vi "SplitString.vi"(8 "error in (no error)":errorcluster, 11 "String in":string) -> (0 "error out":errorcluster, 2 "Array":string[](array[string]), 3 "String out":string)   [LabVIEW 2012]
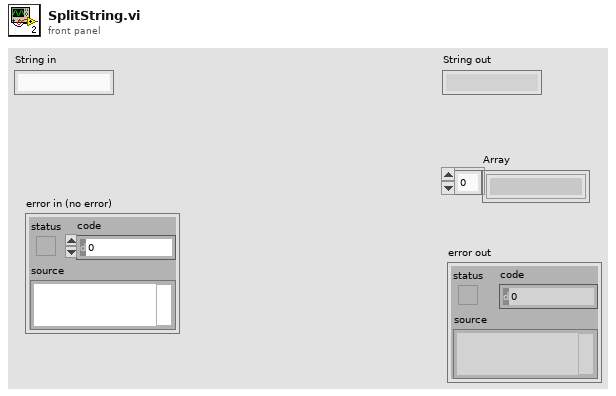
[diagram p1: front panel]
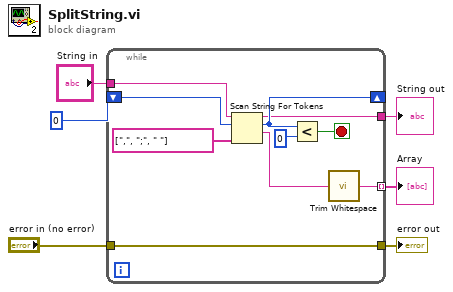
[diagram p0: block diagram]
diagram:
  n1 = while {
    shift-right: [w14] -> _
    shift-left: 0 -> [w16]
    tunnel: "String in" -> [w12]
    tunnel: [w9] -> w3 mode=indexing
    tunnel: "error in (no error)" -> [w8]
    tunnel: [w8] -> w4
    tunnel: [w7] -> w2
    stop <- w13 stop-if-true
    n2 = Scan String For Tokens(6:string[] [",", ";", " "], 8:w16, 9:w12) -> (1:w10:string, 2:w14:i32, 3:w7:string)  [unwired: 3 in, 1 out]
    n3 = Less?(x=w14, y=0) -> (x < y?=w13:bool)
    n4 = call <vilib>:"Trim Whitespace.vi"("string"=w10) -> ("trimmed string"=w9:string)  [unwired: 1 in]
  }
  "String out" <- w2
  "Array" <- w3
  "error out" <- w4
